vi "Hong_experiment_stage_Modified_V2.vi"() -> ()   [LabVIEW 2015]
panel:
  out "MOVE_START_TIME":string
  in  "# of steps":string(combo)
  in  "Step":string(combo)
  out "Step_count":i16
  in  "Load_distance":i32=1000
  out "Load_status":bool=TRUE
  in  "Auto looping":bool=TRUE
  out "msec time 2":u32=742114
  out "msec time 1":u32
  in  "Manual":bool
  out "Scanning":bool=TRUE
  in  "Acc time":u16=100
  in  "Min Scan speed":u32=1000
  in  "Max Scan speed":u32=1500
  in  "Min Initial Speed":u32=1000
  in  "Max Initial Speed":u32=10000
  in  "Res Time":i32=1
  out "Current pos X":i32
  in  "Initail X":i32
  in  "Loop end":i32=10
  out "X pos to move":i32
  in  "Stop":bool
  out "Move OK":bool=TRUE
  in  "Go":bool
  out "Loop cnt":i32=10
  in  "Port number":i8=5
  # "Stage Motion Controller by Gil-Yong Lee 2016. 10. 26. (Ver.1.1) at UW\nModified & Upgraded by Seongheon Hong 2021. 6. 20. (Ver.2.0)"
  # "for the purpose of loading unloading tests (negatice direction control of stage)"
  # "Peak-to-Peak\nunit: um"
  # "Make sure that the COM port set correctly"
  # "unit: um"
  # "Residence time in msec"
  # "unit: um"
  # "unit: um"
  # "Red: Loading, Grey: Unloading"
  # "Speed control"
  # "실제 반복할 때 속도[um/s로 세팅함]. Acc : 100 - 1000 (ms)\nOSMS-26-100 사용시 max : 40000 min : 200"
  # "Shortcutss 1. Go: Page Up 2. Stop: ESC 3. Auto-manual selector: Insert"
  # "Timing monitor"
  # "Operation mode selector"
  # "** Important: Max speed > Min speed"
  # "Note: SGSP step motorized stage with SHOT-702 (Baud rate 38400)"
  # "Max. and Min. speed during process should be carefully controlled\nAcc time smaller than ~ 10 um/s^2 cause malfucntion\nMax speed 90 mm/sec\n(acc time 100, max 90000, min 1000) works (9/4/2015)\n: 10mm/sec ~ 40mm/sec\nMax speed 500 mm/sec (*max HW speed)\n(acc time 1000, max 500000, min 1000) works (9/4/2015)\nTry to increase acc time to increase max speed"
  # "Auto"
  # "Manual"
  # "Max. and Min. speed to initial X Y pos. unit: um/sec"
  # "Port number 7 = COM8"
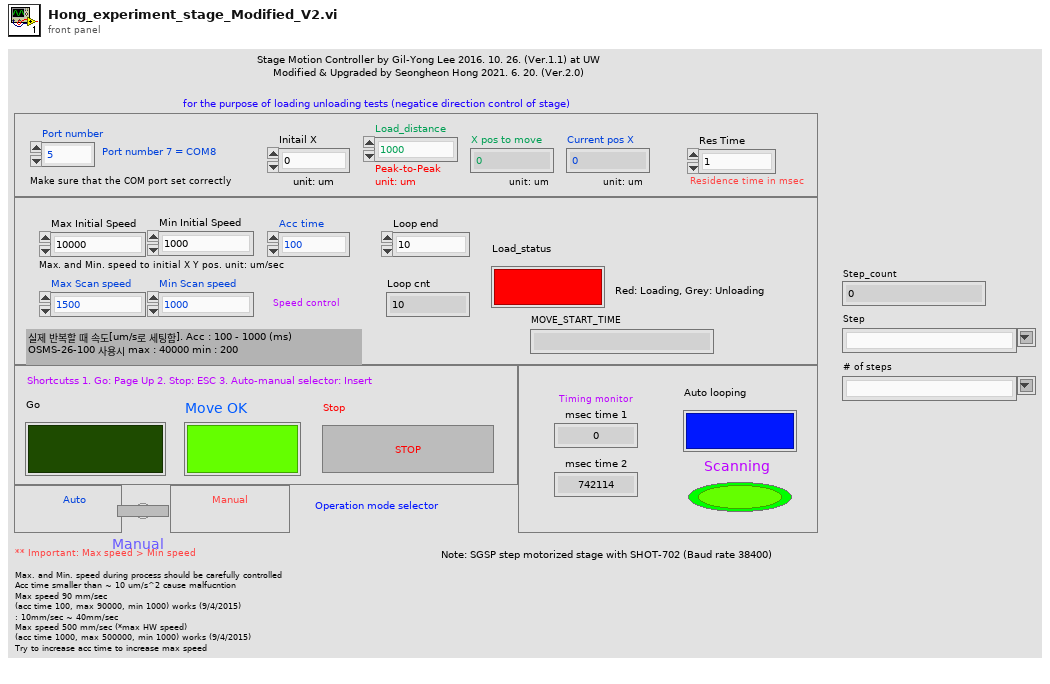
[diagram p1: front panel]
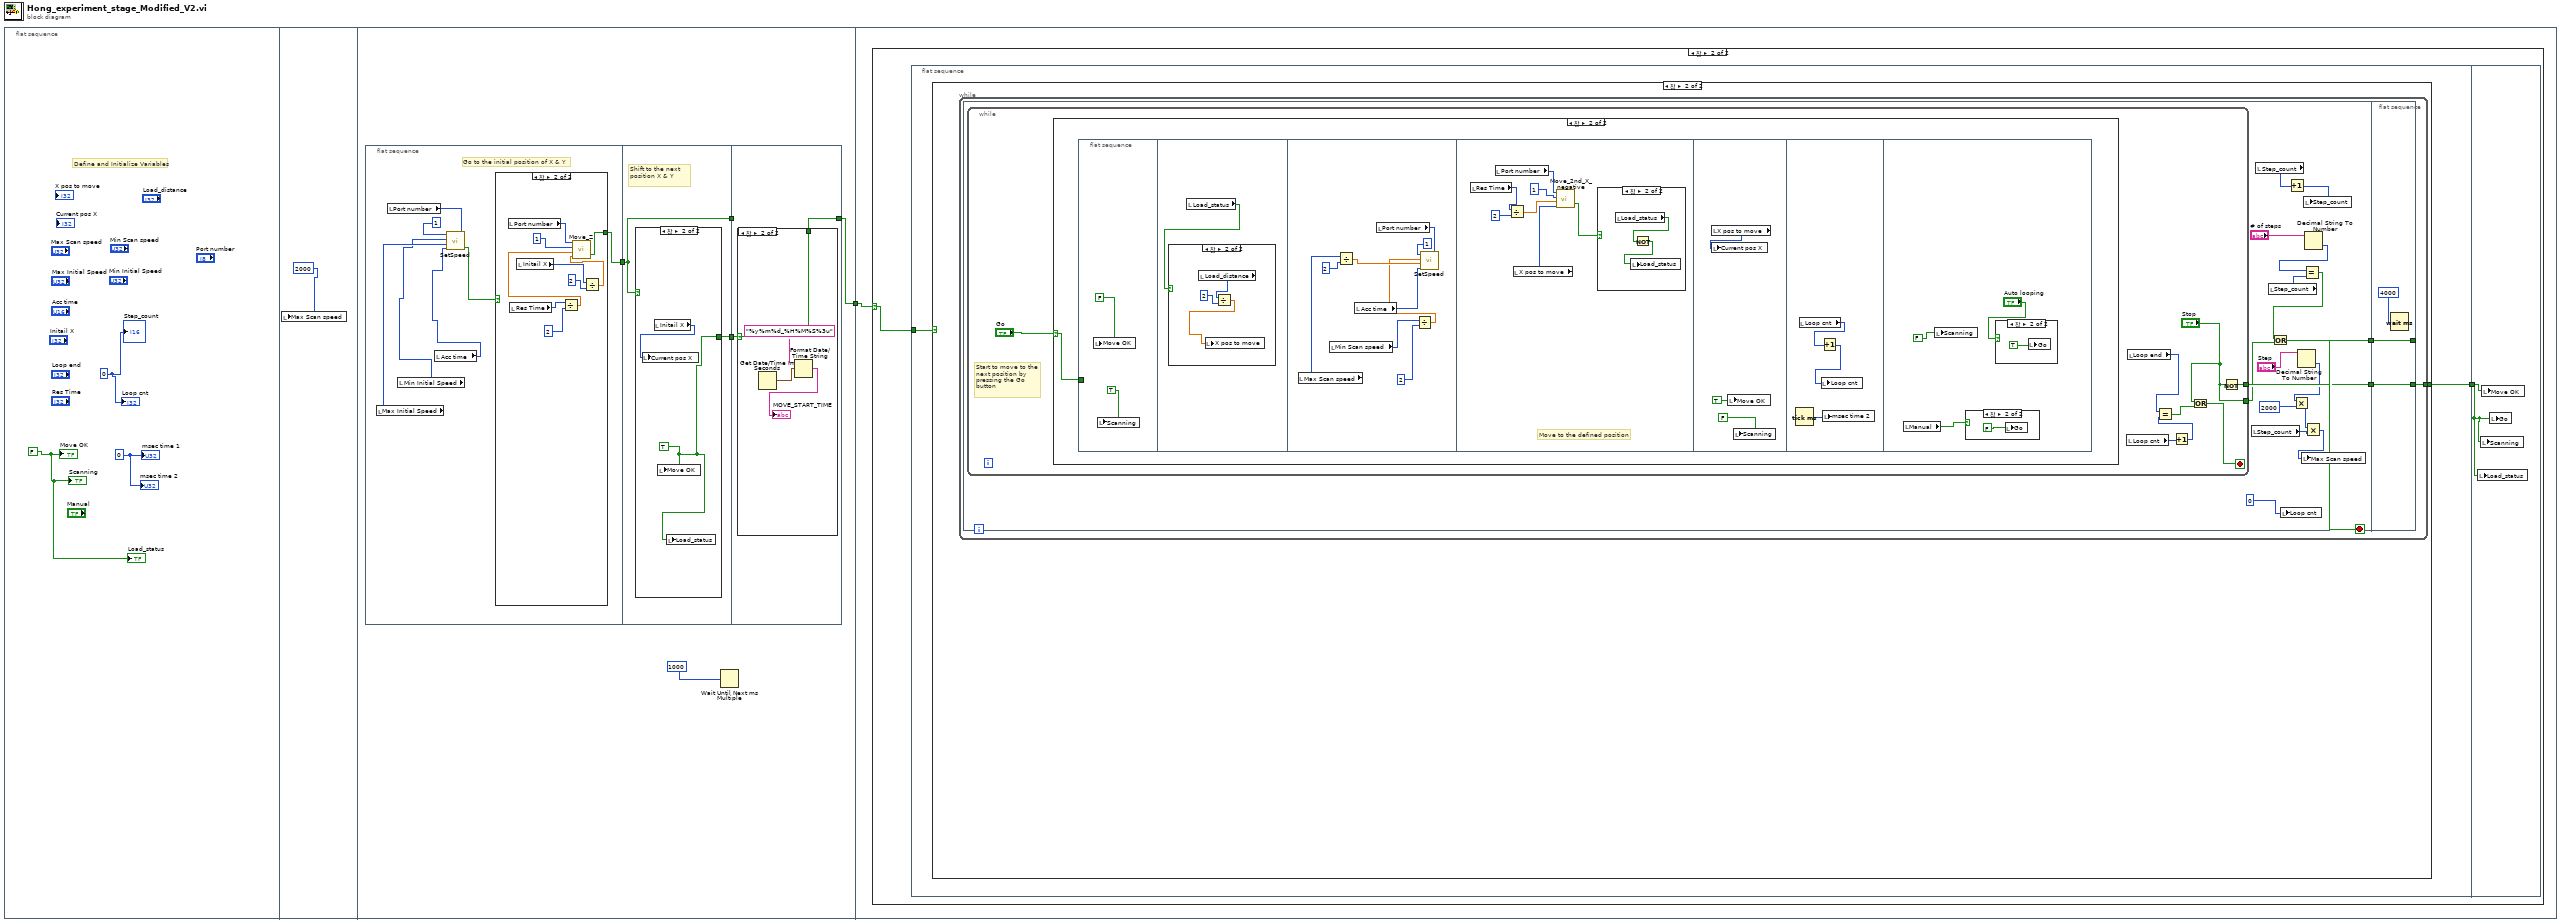
[diagram p0: block diagram]
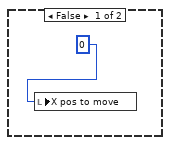
[diagram p8: hidden frame]
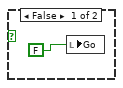
[diagram p10: hidden frame]
diagram:
  n1 = flat-sequence {
    tunnel: [w9] -> w1
    tunnel: w1 -> [w40]
    frame #0 {
      w4 = u32 0
      w3 = FALSE
      w2 = 0
      # "Define and Initialize Variables"
      "Move OK" <- w3
      "Loop cnt" <- w2
      "Scanning" <- w3
      "msec time 1" <- w4
      "msec time 2" <- w4
      "Load_status" <- w3
      "Step_count" <- w2
    }
    frame #1 {
      n2 = local write "Max Scan speed"(2000) -> ()
    }
    frame #2 {
      n3 = flat-sequence {
        tunnel: [w17] -> w10
        tunnel: w10 -> [w29]
        tunnel: [w29] -> w7
        tunnel: [w28] -> w6
        tunnel: [w33] -> w9
        tunnel: w7 -> [_]
        tunnel: w6 -> [w34]
        frame #0 {
          # "Go to the initial position of X & Y"
          n4 = local read "Max Initial Speed"() -> (w14:u32)
          n5 = local read "Port number"() -> (w15:i8)
          n6 = local read "Min Initial Speed"() -> (w13:u32)
          n7 = local read "Acc time"() -> (w12:u16)
          n8 = call "SetSpeed.vi"("Port Number"=w15, "Acceleration Time"=w12, "High Speed"=w14, "Low Speed"=w13, "Axis Number"=u8 1) -> ("OK Done"=w11:bool)  [unwired: 1 out]
          n9 = case shown="참" w11 {
            selector: w11 -> [w18 _]
            tunnel: [w18 w26] -> w17
            frame False {
            }
            frame True {
              n10 = local read "Port number"() -> (w27:i8)
              n11 = local read "Res Time"() -> (w22:i32)
              n12 = local read "Initail X"() -> (w20:i32)
              n13 = Divide(x=w22, y=2) -> (x/y=w23:dbl)
              n14 = Divide(x=w20, y=2) -> (x/y=w19:dbl)
              n15 = call "Move_Z.vi"("Pulse Number"=w19, "Residence time"=w23, "Axis Number"=u8 1, "Port Number Z"=w27) -> ("OK Done"=w26:bool)  [unwired: 1 out]
            }
          }
        }
        frame #1 {
          # "Shift to the next position X & Y"
          n16 = case shown="참" w29 {
            selector: w29 -> [w30 _]
            tunnel: [w30 w31] -> w28
            frame False {
            }
            frame True {
              w31 = TRUE
              n17 = local read "Initail X"() -> (w32:i32)
              n18 = local write "Current pos X"(w32) -> ()
              n19 = local write "Move OK"(w31) -> ()
              n20 = local write "Load_status"(w31) -> ()
            }
          }
        }
        frame #2 {
          n21 = case shown="참" w34 {
            selector: w34 -> [w35 w39]
            tunnel: [w35 w39] -> w33
            frame False {
            }
            frame True {
              n22 = Get Date/Time In Seconds() -> (seconds since 1Jan1904=w38:timestamp)
              n23 = Format Date/Time String(time format string (%c)="%y%m%d_%H%M%S%3u", seconds (now)=w38) -> (date/time string=→"MOVE_START_TIME":string)  [unwired: 1 in]
            }
          }
        }
      }
      n24 = Wait Until Next ms Multiple(millisecond multiple=1000) -> ()  [unwired: 1 out]
    }
    frame #3 {
      n25 = case shown="참" w40 {
        selector: w40 -> [_ w41]
        frame False {
        }
        frame True {
          n26 = flat-sequence {
            tunnel: [w44] -> w42
            tunnel: w41 -> [w43]
            tunnel: w42 -> [w116]
            frame #0 {
              n27 = case shown="참" w43 {
                selector: w43 -> [w45 _]
                tunnel: [w45 w46] -> w44
                frame False {
                }
                frame True {
                  n28 = while {
                    tunnel: [w50] -> w46
                    stop <- w49 stop-if-true
                    n29 = flat-sequence {
                      tunnel: [w66] -> w48
                      tunnel: [w59] -> w47
                      tunnel: [w114] -> w49
                      tunnel: [w115] -> w50
                      tunnel: w48 -> [w115]
                      tunnel: w47 -> [w114]
                      frame #0 {
                        n30 = while {
                          tunnel: [w73] -> w66
                          tunnel: ["Stop"] -> w60
                          stop <- w72 stop-if-true
                          # "Start to move to the next position by pressing the Go button"
                          n31 = case shown="참" "Go" {
                            selector: "Go" -> [_ w75]
                            frame False {
                            }
                            frame True {
                              n32 = flat-sequence {
                                tunnel: w75 -> [_]
                                frame #0 {
                                n33 = local write "Move OK"(FALSE) -> ()
                                n34 = local write "Scanning"(TRUE) -> ()
                                }
                                frame #1 {
                                n35 = local read "Load_status"() -> (w78:bool)
                                n36 = case shown="참" w78 {
                                frame False {
                                n37 = local write "X pos to move"(0) -> ()
                                }
                                frame True {
                                n38 = local read "Load_distance"() -> (w82:i32)
                                n39 = Divide(x=w82, y=2) -> (x/y=w80:dbl)
                                n40 = local write "X pos to move"(w80) -> ()
                                }
                                }
                                }
                                frame #2 {
                                n41 = local read "Max Scan speed"() -> (w88:u32)
                                n42 = local read "Min Scan speed"() -> (w84:u32)
                                n43 = Divide(x=w88, y=2) -> (x/y=w86:dbl)
                                n44 = local read "Acc time"() -> (w89:u16)
                                n45 = local read "Port number"() -> (w90:i8)
                                n46 = Divide(x=w84, y=2) -> (x/y=w83:dbl)
                                n47 = call "SetSpeed.vi"("Port Number"=w90, "Acceleration Time"=w89, "High Speed"=w86, "Low Speed"=w83, "Axis Number"=u8 1) -> ()  [unwired: 2 out]
                                }
                                frame #3 {
                                # "Move to the defined position"
                                n48 = local read "Res Time"() -> (w93:i32)
                                n49 = local read "Port number"() -> (w98:i8)
                                n50 = Divide(x=w93, y=2) -> (x/y=w92:dbl)
                                n51 = local read "X pos to move"() -> (w97:i32)
                                n52 = call "Move_2nd_X_negative.vi"("Pulse Number"=w97, "Residence time"=w92, "Axis Number"=u8 1, "Port Number Z"=w98) -> ("OK Done"=w96:bool)  [unwired: 1 out]
                                n53 = case shown="참" w96 {
                                frame False {
                                }
                                frame True {
                                n54 = local read "Load_status"() -> (w100:bool)
                                n55 = Not(x=w100) -> (.not. x?=w99:bool)
                                n56 = local write "Load_status"(w99) -> ()
                                }
                                }
                                }
                                frame #4 {
                                n57 = local read "X pos to move"() -> (w103:i32)
                                n58 = local write "Current pos X"(w103) -> ()
                                n59 = local write "Move OK"(TRUE) -> ()
                                n60 = local write "Scanning"(FALSE) -> ()
                                }
                                frame #5 {
                                n61 = Tick Count (ms)() -> (millisecond timer value=w104:u32)
                                n62 = local read "Loop cnt"() -> (w106:i32)
                                n63 = Increment(x=w106) -> (x+1=w105:i32)
                                n64 = local write "Loop cnt"(w105) -> ()
                                n65 = local write "msec time 2"(w104) -> ()
                                }
                                frame #6 {
                                n66 = local read "Manual"() -> (w109:bool)
                                n67 = local write "Scanning"(FALSE) -> ()
                                n68 = case shown="참" w109 {
                                frame False {
                                }
                                frame True {
                                n69 = local write "Go"(FALSE) -> ()
                                }
                                }
                                n70 = case shown="참" "Auto looping" {
                                frame False {
                                n71 = local write "Go"(FALSE) -> ()
                                }
                                frame True {
                                n72 = local write "Go"(TRUE) -> ()
                                }
                                }
                                }
                              }
                            }
                          }
                          n73 = local read "Loop cnt"() -> (w69:i32)
                          n74 = local read "Loop end"() -> (w71:i32)
                          n75 = Increment(x=w69) -> (x+1=w68:i32)
                          n76 = Equal?(x=w71, y=w68) -> (x = y?=w70:bool)
                          n77 = Or(x="Stop", y=w70) -> (x .or. y?=w72:bool)
                          n78 = Not(x="Stop") -> (.not. x?=w73:bool)
                        }
                        n79 = local read "Step_count"() -> (w55:i16)
                        n80 = local read "Step_count"() -> (w65:i16)
                        n81 = local read "Step_count"() -> (w62:i16)
                        n82 = local write "Loop cnt"(0) -> ()
                        n83 = Increment(x=w65) -> (x+1=w64:i16)
                        n84 = Decimal String To Number(string="Step") -> (number=w58:i32)  [unwired: 2 in, 1 out]
                        n85 = Multiply(x=w58, y=2000) -> (x*y=w56:i32)
                        n86 = local write "Step_count"(w64) -> ()
                        n87 = Multiply(x=w56, y=w55) -> (x*y=w54:i32)
                        n88 = local write "Max Scan speed"(w54) -> ()
                        n89 = Decimal String To Number(string="# of steps") -> (number=w63:i32)  [unwired: 2 in, 1 out]
                        n90 = Equal?(x=w63, y=w62) -> (x = y?=w61:bool)
                        n91 = Or(x=w61, y=w60) -> (x .or. y?=w59:bool)
                      }
                      frame #1 {
                        n92 = Wait (ms)(milliseconds to wait=4000) -> ()  [unwired: 1 out]
                      }
                    }
                  }
                }
              }
            }
            frame #1 {
              n93 = local write "Load_status"(w116) -> ()
              n94 = local write "Scanning"(w116) -> ()
              n95 = local write "Move OK"(w116) -> ()
              n96 = local write "Go"(w116) -> ()
            }
          }
        }
      }
    }
  }
